vi "Start Scan.vi"(8 "error in (no error)":errorcluster, 10 "Scan Settings":T1, 11 "Context in":refnum<class "Context.lvclass">) -> (0 "error out":errorcluster, 3 "Context out":refnum<class "Context.lvclass">)   [LabVIEW 2015, in "Context.lvclass"]
uses:
  Context.lvclass
  Model/Model/Model.lvclass
  States/State/State.lvclass
  Typedefs/ScanSettings.ctl
  Typedefs/FAMT Typedefs.lvlib
  Typedefs/WaveformTypes.ctl
  Typedefs/WaveformSettings.ctl
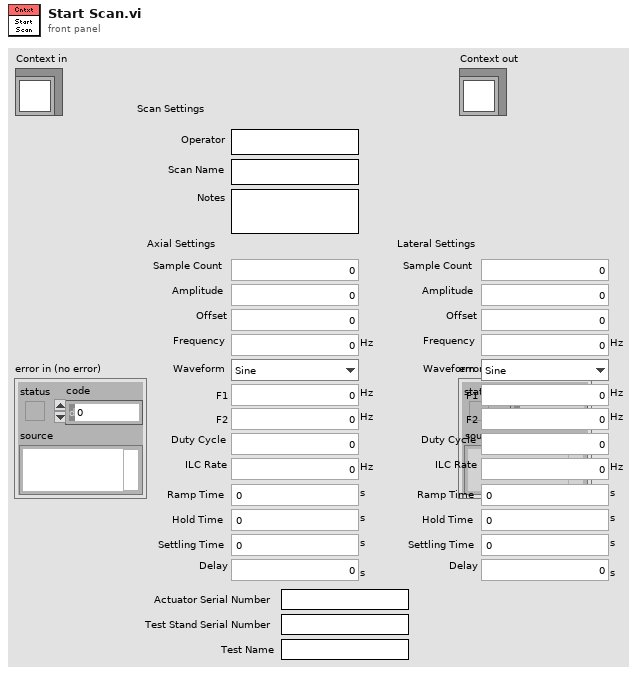
[diagram p1: front panel]
types:
  T1 = typedef "FAMT Typedefs.lvlib/ScanSettings.ctl" = cluster{"Operator":string, "Scan Name":string, "Notes":string, "Axial Settings":T2, "Lateral Settings":T2, "Actuator Serial Number":string, "Test Stand Serial Number":string, "Test Name":string}
  T2 = typedef "FAMT Typedefs.lvlib/WaveformSettings.ctl" = cluster{"Sample Count":u32, "Amplitude":dbl, "Offset":dbl, "Frequency":dbl[unit], "Waveform":T3, "F1":dbl[unit], "F2":dbl[unit], "Duty Cycle":dbl, "ILC Rate":dbl[unit], "Ramp Time":dbl[unit], "Hold Time":dbl[unit], "Settling Time":dbl[unit], "Delay":dbl[unit]}
  T3 = typedef "FAMT Typedefs.lvlib/WaveformTypes.ctl" = enum16{"Sine", "Triangle", "Square", "Sawtooth", "Chirp", "Gaussian", "Trapezoid", "Constant"}
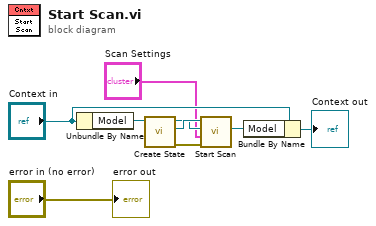
[diagram p0: block diagram]
diagram:
  n1 = Unbundle By Name("Context in") -> ("Model"=w8:refnum<class "Model.lvclass">)
  n2 = call "Create State.vi"("Model in"=w8) -> ("error out"=w2:errorcluster, "State"=w4:refnum<class "State.lvclass">, "Model out"=w3:refnum<class "Model.lvclass">)  [unwired: 8 in]
  n3 = call-dynamic "Start Scan.vi"("error in (no error)"=w2, "Scan Settings"="Scan Settings", "Model in"=w3, "State in"=w4) -> ("Model out"=w5:refnum<class "Model.lvclass">)  [unwired: 5 in, 2 out]
  n4 = Bundle By Name(cluster="Context in", "Model"=w5) -> (→"Context out":refnum<class "Context.lvclass">)
  "error out" <- "error in (no error)"
